vi "Initialize.vi"(8 "error in (no error)":errorcluster, 9 "Reset (True)":bool=TRUE, 10 "ID Query (True)":bool=TRUE, 11 "VISA resource name":refnum<visa-resource-name>) -> (0 "error out":errorcluster, 3 "VISA resource name out":refnum<visa-resource-name>)   [LabVIEW 2019, in "Agilent 2000 3000 X-Series.lvlib"]
doc: "Establishes communication with the instrument and optionally performs an instrument identification query and/or an instrument reset. It also places the instrument in a default state needed for other instrument driver operations. Therefore, call this VI before calling other instrument driver VIs for this instrument. Generally, you need to call the Initialize VI only once at the beginning of an application."
uses:
  Agilent 2000 3000 X-Series.lvlib
  Private/Extended User Data.ctl
panel:
  # "(c) 2011-2013 National Instruments.  ALL RIGHTS RESERVED."
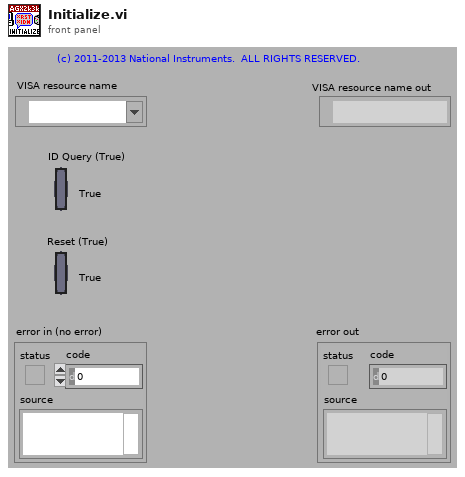
[diagram p1: front panel]
types:
  T1 = typedef "Agilent 2000 3000 X-Series.lvlib/Extended User Data.ctl" = cluster{"X-Series Mode":u16, "Acquisition Type (0: Normal)":i32}
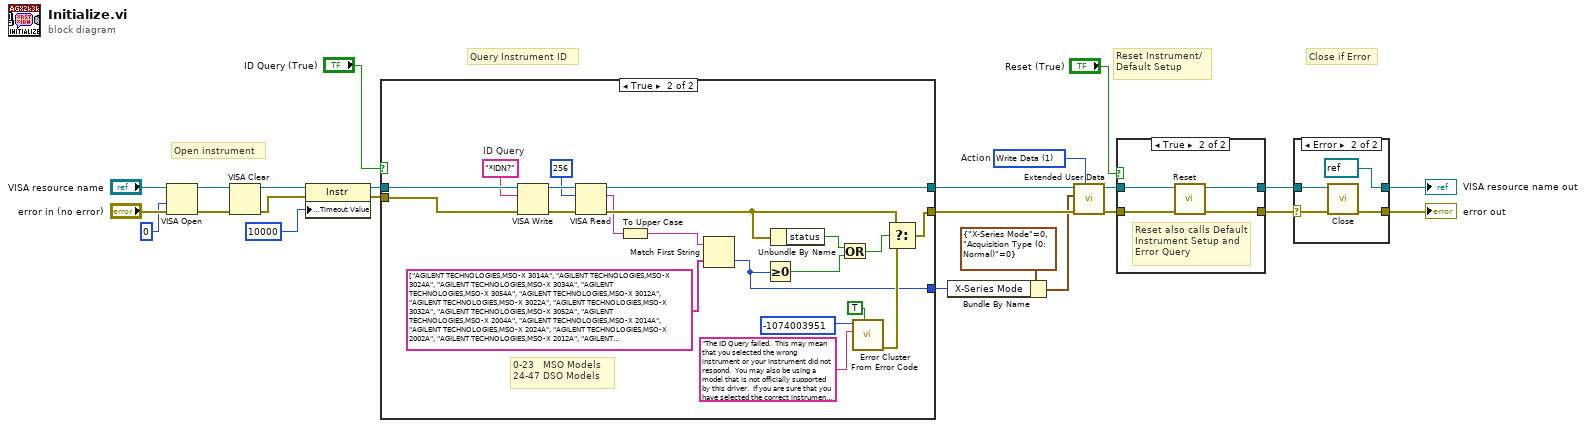
[diagram p0: block diagram]
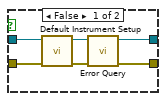
[diagram p3: hidden frame]
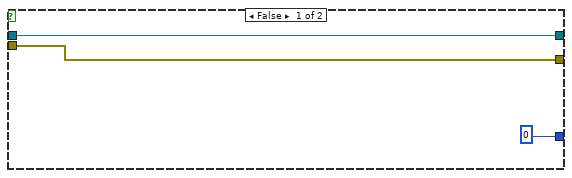
[diagram p4: hidden frame]
diagram:
  w8 = 1 items=["Read Data", "Write Data", "Clear Data", "Clear ALL Data"]  # Action
  # "Close if Error"
  # "Query Instrument ID"
  # "Reset Instrument/\nDefault Setup"
  # "Open instrument"
  n1 = VISA Open(access mode=u32 0, error in (no error)="error in (no error)", VISA resource name="VISA resource name") -> (VISA resource name=w18:refnum<visa-resource-name>, error out=w17:errorcluster)  [unwired: 2 out]
  n2 = VISA Clear(VISA resource name=w18, error in (no error)=w17) -> (VISA resource name out=w16:refnum<visa-resource-name>, error out=w15:errorcluster)
  n3 = property class="Instr"(reference=w16, error in=w15, "General Settings:Timeout Value"=u32 10000) -> (reference out=w10:refnum<visa-resource-name>, error out=w9:errorcluster)
  n4 = case shown="True" "ID Query (True)" {
    tunnel: [w26 w47] -> w5
    tunnel: [w27 w45] -> w7
    tunnel: w10 -> [w27 w46]
    tunnel: w9 -> [w26 w32]
    tunnel: [u16 0 ("X-Series Mode") w31] -> w1
    frame False {
    }
    frame True {
      w41 = "*IDN?"  # ID Query
      # "0-23   MSO Models\n24-47 DSO Models"
      n5 = VISA Write(VISA resource name=w46, write buffer=w41, error in (no error)=w32) -> (VISA resource name out=w44:refnum<visa-resource-name>, error out=w43:errorcluster)  [unwired: 1 out]
      n6 = VISA Read(VISA resource name=w44, byte count=u32 256, error in (no error)=w43) -> (VISA resource name out=w45:refnum<visa-resource-name>, read buffer=w30:string, error out=w36:errorcluster)  [unwired: 1 out]
      n7 = To Upper Case(1:w30) -> (0:w29:string)
      n8 = Match First String(2:string[] ["AGILENT TECHNOLOGIES,MSO-X 3014A", "AGILENT TECHNOLOGIES,MSO-X 3024A", "AGILENT TECHNOLOGIES,MSO-X 3034A", "AGILENT TECHNOLOGIES,MSO-X 3054A", "AGILENT TECHNOLOGIES,MSO-X 3012A", "AGILENT TECHNOLOGIES,MSO-X 3022A", "AGILENT TECHNOLOGIES,MSO-X 3032A", "AGILENT TECHNOLOGIES,MSO-X 3052A", "AGILENT TECHNOLOGIES,MSO-X 2004A", "AGILENT TECHNOLOGIES,MSO-X 2014A", "AGILENT TECHNOLOGIES,MSO-X 2024A", "AGILENT TECHNOLOGIES,MSO-X 2002A", "AGILENT TECHNOLOGIES,MSO-X 2012A", "AGILENT TECHNOLOGIES,MSO-X 2022A", "AGILENT TECHNOLOGIES,MSO-X 3104A", "AGILENT TECHNOLOGIES,MSO-X 3102A", "AGILENT TECHNOLOGIES,MSO-X 4154A", "AGILENT TECHNOLOGIES,MSO-X 4104A", "AGILENT TECHNOLOGIES,MSO-X 4054A", "AGILENT TECHNOLOGIES,MSO-X 4034A", "AGILENT TECHNOLOGIES,MSO-X 4024A", "AGILENT TECHNOLOGIES,MSO-X 4052A", "AGILENT TECHNOLOGIES,MSO-X 4032A", "AGILENT TECHNOLOGIES,MSO-X 4022A", "AGILENT TECHNOLOGIES,DSO-X 3014A", "AGILENT TECHNOLOGIES,DSO-X 3024A", "AGILENT TECHNOLOGIES,DSO-X 3034A", "AGILENT TECHNOLOGIES,DSO-X 3054A", "AGILENT TECHNOLOGIES,DSO-X 3012A", "AGILENT TECHNOLOGIES,DSO-X 3022A", "AGILENT TECHNOLOGIES,DSO-X 3032A", "AGILENT TECHNOLOGIES,DSO-X 3052A", "AGILENT TECHNOLOGIES,DSO-X 2004A", "AGILENT TECHNOLOGIES,DSO-X 2014A", "AGILENT TECHNOLOGIES,DSO-X 2024A", "AGILENT TECHNOLOGIES,DSO-X 2002A", "AGILENT TECHNOLOGIES,DSO-X 2012A", "AGILENT TECHNOLOGIES,DSO-X 2022A", "AGILENT TECHNOLOGIES,DSO-X 3104A", "AGILENT TECHNOLOGIES,DSO-X 3102A", "AGILENT TECHNOLOGIES,DSO-X 4154A", "AGILENT TECHNOLOGIES,DSO-X 4104A", "AGILENT TECHNOLOGIES,DSO-X 4054A", "AGILENT TECHNOLOGIES,DSO-X 4034A", "AGILENT TECHNOLOGIES,DSO-X 4024A", "AGILENT TECHNOLOGIES,DSO-X 4052A", "AGILENT TECHNOLOGIES,DSO-X 4032A", "AGILENT TECHNOLOGIES,DSO-X 4022A"], 3:w29) -> (0:w31:i32)  [unwired: 1 out]
      n9 = Greater Or Equal To 0?(x=w31) -> (x >= 0?=w34:bool)
      n10 = Unbundle By Name(w36) -> ("status"=w35:bool)
      n11 = Or(x=w35, y=w34) -> (x .or. y?=w33:bool)
      n12 = call <vilib>:"Error Cluster From Error Code.vi"("show call chain? (False)"=TRUE, "error message (\"\")"="The ID Query failed.  This may mean that you selected the wrong instrument or your instrument did not respond.  You may also be using a model that is not officially supported by this driver.  If you are sure that you have selected the correct instrument and it is responding, try disabling the ID Query." ("Source (VI Name)"), "error code (0)"=-1074003951 ("Code")) -> ("error out"=w40:errorcluster)  [unwired: 1 in, 5 out]
      n13 = Select(t=w36, s=w33, f=w40) -> (s? t:f=w47:errorcluster)
    }
  }
  n14 = Bundle By Name(cluster=T1 {"X-Series Mode"=0, "Acquisition Type (0: Normal)"=0} ("User Data Definition"), "X-Series Mode"=w1) -> (w3:T1)
  n15 = call "Extended User Data.vi"("Action (1: Write Data)"=w8, "error in (no error)"=w5, "User Data In"=w3, "VISA resource name in"=w7) -> ("error out"=w4:errorcluster, "VISA resource name out"=w6:refnum<visa-resource-name>)  [unwired: 6 out]
  n16 = case shown="True" "Reset (True)" {
    tunnel: w4 -> [w52 w54]
    tunnel: [w49 w57] -> w11
    tunnel: w6 -> [w53 w55]
    tunnel: [w50 w56] -> w12
    frame False {
      n17 = call "Default Instrument Setup.vi"("error in (no error)"=w52, "VISA resource name"=w53) -> ("error out"=w48:errorcluster, "VISA resource name out"=w51:refnum<visa-resource-name>)  [unwired: 8 out]
      n18 = call "Error Query.vi"("error in (no error)"=w48, "VISA resource name"=w51) -> ("error out"=w49:errorcluster, "VISA resource name out"=w50:refnum<visa-resource-name>)  [unwired: 8 out]
    }
    frame True {
      # "Reset also calls Default Instrument Setup and Error Query"
      n19 = call "Reset.vi"("error in (no error)"=w54, "VISA resource name"=w55) -> ("error out"=w57:errorcluster, "VISA resource name out"=w56:refnum<visa-resource-name>)  [unwired: 8 out]
    }
  }
  n20 = case shown="Error" w11 {
    selector: w11 -> [w58 w61]
    tunnel: w12 -> [w59 w62]
    tunnel: [w59 refnum<visa-resource-name> refnum ("VISA resource name out")] -> w14
    tunnel: [w58 w63] -> w13
    frame No Error {
    }
    frame Error {
      n21 = call "Close.vi"("error in (no error)"=w61, "VISA resource name"=w62) -> ("error out"=w63:errorcluster)  [unwired: 9 out]
    }
  }
  "VISA resource name out" <- w14
  "error out" <- w13
